vi "EEUpload.vi"(8 "error in (no error)":errorcluster caption="错误输入（无错误）", 9 "PN":string, 10 "打印模式":enum16{"IT Print", "EE Print"}(ring)=enum."EE Print" caption="Print Mode", 11 "xmlConfigPath":path caption="XML文档路径") -> (0 "错误输出":errorcluster, 2 "EEUPLOAD":bool, 3 "EEUploadPN":string[](array[string]))   [LabVIEW 2011]
uses:
  Data/xmlFunction.dll
  <vilib>/xml/Load XML File.vi
  <vilib>/xml/Close Reference(Node).vi
  <vilib>/xml/NI_XML.lvlib
  C:/Program Files (x86)/National Instruments/LabVIEW 2011/resource/objmgr/DOMUserDefRef.rc
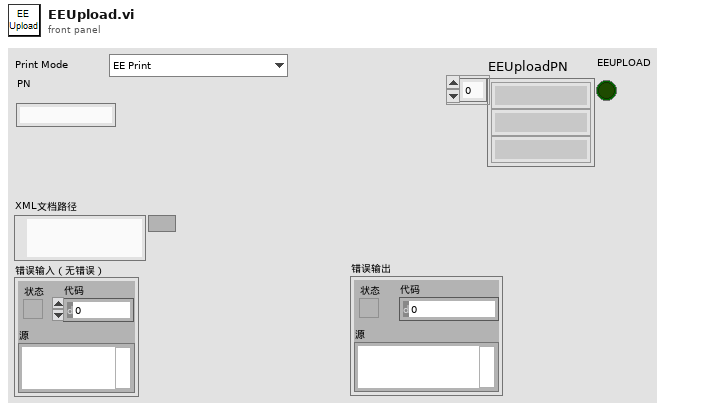
[diagram p1: front panel]
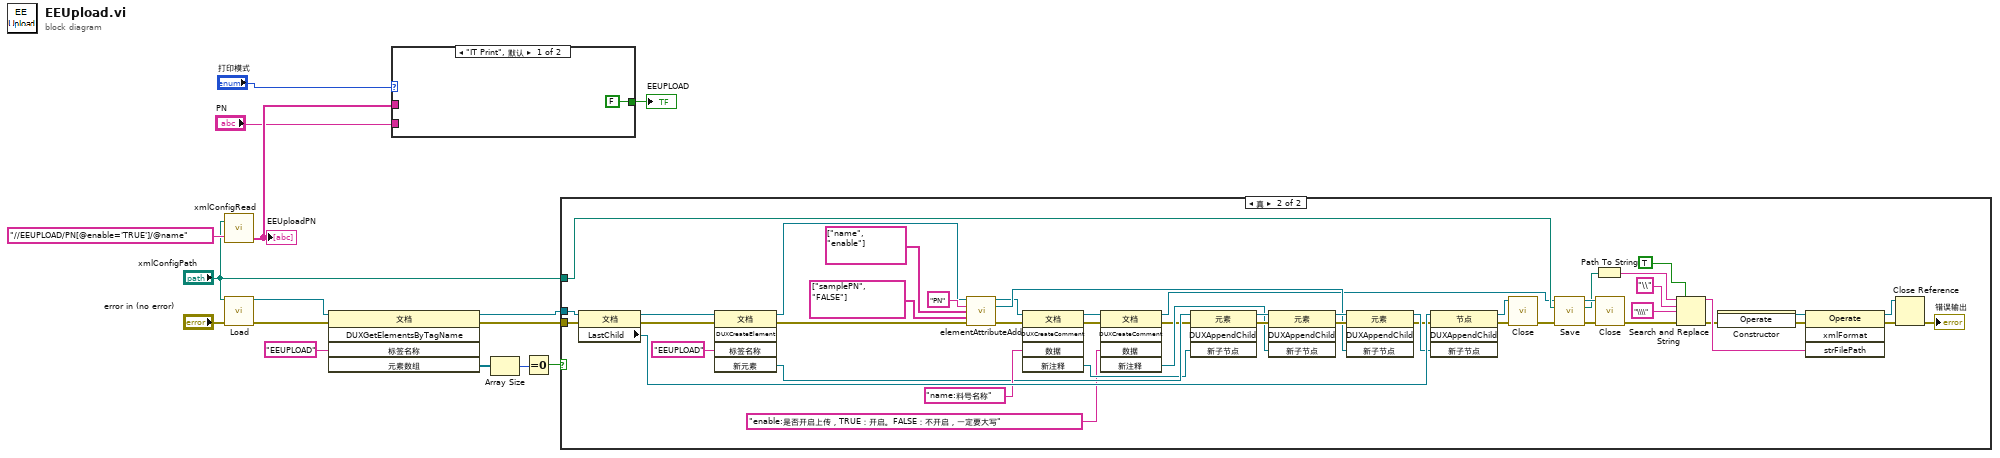
[diagram p0: block diagram]
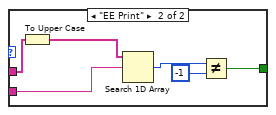
[diagram p2: hidden frame]
diagram:
  n1 = call "xmlConfigRead.vi"("path to XML document"="xmlConfigPath", "XPath expression"="//EEUPLOAD/PN[@enable='TRUE']/@name") -> ("OutParaArray"=w3:string[])  [unwired: 2 out]
  "EEUploadPN" <- w3
  n2 = call-poly <vilib>:"Load.vi"("path to XML document"="xmlConfigPath", "error in (no error)"="error in (no error)") -> ("DOM document out"=w14:refnum<k20>, "error out"=w8:errorcluster)  [unwired: 11 in, 1 out]
  n3 = invoke class="文档" method="DUXGetElementsByTagName"(reference=w14, error in=w8, "标签名称"="EEUPLOAD") -> (reference out=w9:refnum<k20>, error out=w7:errorcluster, "元素数组"=w12:refnum<k20>[])  [unwired: 2 in, 2 out]
  n4 = case shown="\"IT Print\", 默认" "打印模式" {
    tunnel: w3 -> [_ w22]
    tunnel: "PN" -> [_ w20]
    tunnel: [FALSE w17] -> w1
    frame "IT Print", Default {
    }
    frame "EE Print" {
      n5 = To Upper Case(1:w22) -> (0:w21:string[])
      n6 = Search 1D Array(1D array=w21, element=w20) -> (index of element=w19:i32)  [unwired: 1 in]
      n7 = Not Equal?(x=w19, y=-1) -> (x != y?=w17:bool)
    }
  }
  "EEUPLOAD" <- w1
  n8 = Array Size(array=w12) -> (size(s)=w11:i32)
  n9 = Equal To 0?(x=w11) -> (x = 0?=w10:bool)
  n10 = case shown="真" w10 {
    tunnel: "xmlConfigPath" -> [_ w70]
    tunnel: w7 -> [_ w45]
    tunnel: w9 -> [_ w34]
    frame False {
    }
    frame True {
      n11 = property class="文档"(reference=w34, error in=w45) -> (reference out=w68:refnum<k20>, error out=w66:errorcluster, "LastChild"=w69:refnum<k20>)
      n12 = invoke class="文档" method="DUXCreateElement"(reference=w68, error in=w66, "标签名称"="EEUPLOAD") -> (reference out=w40:refnum<k20>, error out=w37:errorcluster, "新元素"=w55:refnum<k20>)  [unwired: 2 in, 2 out]
      n13 = call "elementAttributeAdd.vi"("DOM document in"=w40, "elementName"="PN" ("标签名称"), "property"=string[] ["name", "enable"], "value"=string[] ["samplePN", "FALSE"], "错误输入（无错误）"=w37) -> ("DOM document out"=w26:refnum<k20>, "element"=w35:refnum<k20>, "错误输出"=w25:errorcluster)  [unwired: 8 in]
      n14 = invoke class="文档" method="DUXCreateComment"(reference=w26, error in=w25, "数据"="name:料号名称") -> (reference out=w50:refnum<k20>, error out=w47:errorcluster, "新注释"=w54:refnum<k20>)  [unwired: 2 in, 2 out]
      n15 = invoke class="文档" method="DUXCreateComment"(reference=w50, error in=w47, "数据"="enable:是否开启上传，TRUE：开启。FALSE：不开启，一定要大写") -> (reference out=w27:refnum<k20>, error out=w46:errorcluster, "新注释"=w48:refnum<k20>)  [unwired: 2 in, 2 out]
      n16 = invoke class="元素" method="DUXAppendChild"(reference=w55, error in=w46, "新子节点"=w54) -> (reference out=w53:refnum<k20>, error out=w51:errorcluster)  [unwired: 1 in, 2 out]
      n17 = invoke class="元素" method="DUXAppendChild"(reference=w53, error in=w51, "新子节点"=w48) -> (reference out=w52:refnum<k20>, error out=w36:errorcluster)  [unwired: 1 in, 2 out]
      n18 = invoke class="元素" method="DUXAppendChild"(reference=w52, error in=w36, "新子节点"=w35) -> (reference out=w24:refnum<k20>, error out=w23:errorcluster)  [unwired: 1 in, 2 out]
      n19 = invoke class="节点" method="DUXAppendChild"(reference=w69, error in=w23, "新子节点"=w24) -> (reference out=w56:refnum<k20>, error out=w33:errorcluster)  [unwired: 1 in, 2 out]
      n20 = call-poly <vilib>:"Close.vi"("error in (no error)"=w33, "node"=w56) -> ("error out"=w32:errorcluster)  [unwired: 7 out]
      n21 = call <vilib>:"Save.vi"("error in (no error)"=w32, "XML file path"=w70, "DOM document in"=w27) -> ("error out"=w30:errorcluster, "XML file path out"=w28:path, "DOM document out"=w31:refnum<k20>)  [unwired: 6 in]
      n22 = Path To String(path=w28) -> (string=w65:string)
      n23 = call-poly <vilib>:"Close.vi"("error in (no error)"=w30, "node"=w31) -> ("error out"=w29:errorcluster)  [unwired: 7 in]
      n24 = Search and Replace String(replace all?=TRUE ("替换全部？(F)"), input string=w65, search string="\\" ("搜索字符串"), replace string="\\\\" ("替换字符串(\"\")"), error in=w29) -> (result string=w60:string, error out=w58:errorcluster)  [unwired: 3 in, 2 out]
      n25 = constructor class="Operate"(error in=w58) -> (reference out=w61:refnum<k24>, error out=w59:errorcluster)  [unwired: 2 in, 1 out]
      n26 = invoke class="Operate" method="xmlFormat"(reference=w61, error in=w59, "strFilePath"=w60) -> (reference out=w44:refnum<k24>, error out=w43:errorcluster)  [unwired: 1 in, 2 out]
      n27 = Close Reference(reference=w44, error in (no error)=w43) -> (error out=→"错误输出":errorcluster)
    }
  }
